vi "SMART__Yt12_GenericTest.vi"() -> ()   [LabVIEW 2017]
uses:
  Step`s VIs/YYLLIdea/yylltestresult/yylltestresult basis.ctl
  <vilib>/Utility/miscctls.llb/LVPointTypeDef.ctl
panel:
  in  "Bool数据源":bool
  out "数据源预览":string
  in  "Smart预处理":string[][](array[string])
  in  "数据源什么类型？":enum16{"String类型", "NUM类型", "Bool类型"}(ring)
  in  "String数据源":string
  out "预处理后文本":string
  in  "Smart发送预处理btn":bool
  in  "NUM数据源":dbl
  out "结果预览":bool
  in  "LowLimit-C":dbl
  in  "UpperLimit-B":dbl
  in  "StringLimit-A":string
  in  "合格依据":T1 caption="Enum 3"
  # "#yylltips:要判断MAC可以通过正则“\\w{12}”"
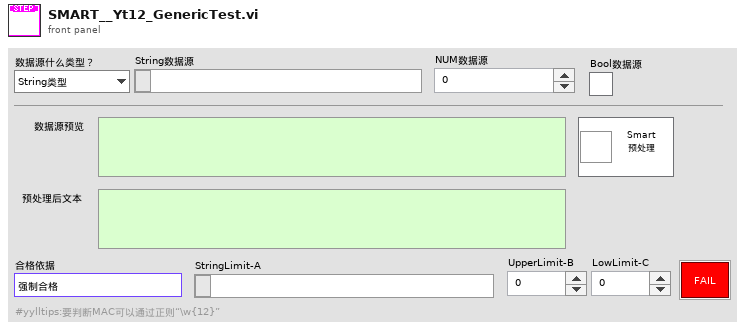
[diagram p1: front panel]
types:
  T1 = typedef "yylltestresult basis.ctl" = enum16{"强制合格", "强制不合格", "随机合格", "X=A", "X=\"真\"", "X=\"假\"", "X≠A", "X包含A", "X不包含A", "A包含X", "A包含非空X", "A不包含X", "X等于A正则匹配内容", "X包含A正则匹配内容", "X不包含A正则匹配内容", "X=B", "X≠B", "X＞B", "X≥B", "X＜B", "X≤B", "B≥X≥C", "B≥X＞C", "B＞X≥C", "B＞X＞C", "X≥B | C≥X", "X＞B | C≥X", "X≥B | C＞X", "X＞B | C＞X"}
  T2 = typedef "LVPointTypeDef.ctl" = cluster{"Horizontal":i16, "Vertical":i16}
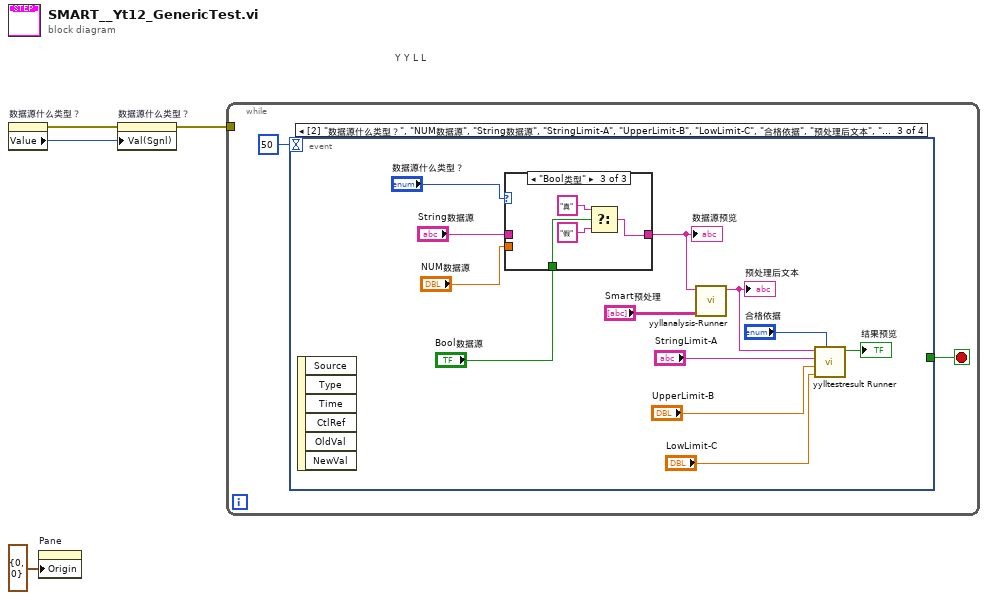
[diagram p0: block diagram]
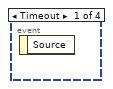
[diagram p2: hidden frame]
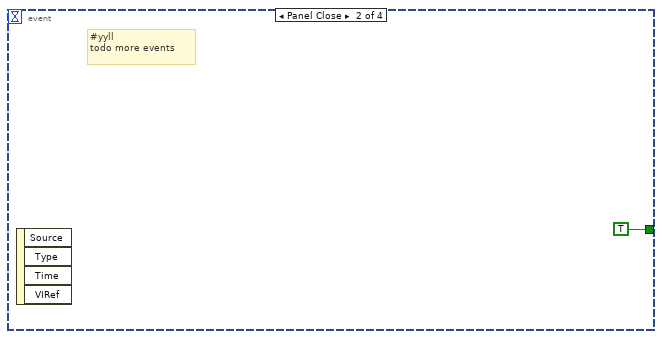
[diagram p3: hidden frame]
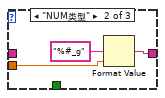
[diagram p5: hidden frame]
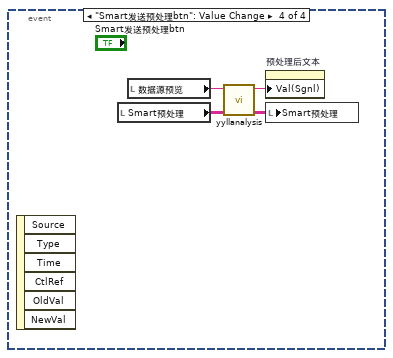
[diagram p6: hidden frame]
diagram:
  # "Y Y L L"
  n1 = property on="数据源什么类型？" class="Enum (strict)"() -> (error out=w1:errorcluster, "Value"=w3:enum16{"String类型", "NUM类型", "Bool类型"})  [unwired: 2 in, 1 out]
  n2 = property on="Pane" class="Pane"("Origin"=T2 {"Horizontal"=0, "Vertical"=0}) -> ()  [unwired: 2 in, 2 out]
  n3 = property on="数据源什么类型？" class="Enum (strict)"(error in=w1, "Val(Sgnl)"=w3) -> (error out=w2:errorcluster)  [unwired: 1 in, 1 out]
  n4 = while {
    tunnel: w2 -> [_]
    stop <- w5 stop-if-true
    n5 = event shown="[2] \"数据源什么类型？\", \"NUM数据源\", \"String数据源\", \"StringLimit-A\", \"UpperLimit-B\", \"LowLimit-C\", \"合格依据\", \"预处理后文本\", \"Bool数据源\": Value Change" {
      selector: _ -> [_ _ _ _]
      dyn-events: _ -> [_ _ _ _]
      timeout: 50 -> [_ _ _ _]
      tunnel: [_ TRUE ("Discard?") _ _] -> w5
      event Timeout {
        n6 = event-data() -> ()  [unwired: 1 in, 1 out]
      }
      event Panel Close {
        # "#yyll\ntodo more events"
        n7 = event-data() -> ()  [unwired: 1 in, 4 out]
      }
      event "数据源什么类型？", "NUM数据源", "String数据源", "StringLimit-A", "UpperLimit-B", "LowLimit-C", "预处理后文本", "Bool数据源": Value Change {
        n8 = event-data() -> ()  [unwired: 1 in, 6 out]
        n9 = case shown="\"Bool类型\"" "数据源什么类型？" {
          tunnel: "String数据源" -> [w20 _ _]
          tunnel: [w20 w22 w24] -> w14
          tunnel: "NUM数据源" -> [_ w23 _]
          tunnel: "Bool数据源" -> [_ _ w25]
          frame "String类型" {
          }
          frame "NUM类型" {
            n10 = Format Value(format string="%#_g", value (0)=w23) -> (output string=w22:string)  [unwired: 1 in]
          }
          frame "Bool类型" {
            n11 = Select(t="真", s=w25, f="假") -> (s? t:f=w24:string)
          }
        }
        "数据源预览" <- w14
        n12 = call "yyllanalysis-Runner.vi"("inputs"="Smart预处理", "String in"=w14) -> ("String out"=w15:string)  [unwired: 8 in, 1 out]
        "预处理后文本" <- w15
        n13 = call "yylltestresult Runner.vi"("合格依据"="合格依据", "LowLimit-C"="LowLimit-C", "UpperLimit-B"="UpperLimit-B", "StringLimit-A"="StringLimit-A", "DataIn-X"=w15) -> ("isPass"=→"结果预览":bool)  [unwired: 4 in, 2 out]
      }
      event "Smart发送预处理btn": Value Change {
        n14 = event-data() -> ()  [unwired: 1 in, 6 out]
        n15 = local read "Smart预处理"() -> (w31:string[][])
        n16 = local read "数据源预览"() -> (w29:string)
        n17 = call "yyllanalysis.vi"("Datain"=w31, "StringIN"=w29) -> ("Dataout"=w30:string[][], "StringOUT"=w28:string)  [unwired: 8 in]
        n18 = property on="预处理后文本" class="Str"("Val(Sgnl)"=w28) -> ()  [unwired: 2 in, 2 out]
        n19 = local write "Smart预处理"(w30) -> ()
      }
    }
  }
